vi "run.vi"(8 "error in (no error)":errorcluster, 11 "canon_m3 in":refnum<class "protocol_canonM3.lvclass">) -> (0 "error out":errorcluster, 3 "canon_m3 out":refnum<class "protocol_canonM3.lvclass">)   [LabVIEW 2015, in "protocol_canonM3.lvclass"]
uses:
  protocol_canonM3.lvclass
  protocol_Generic/Protocol_Generic.lvclass
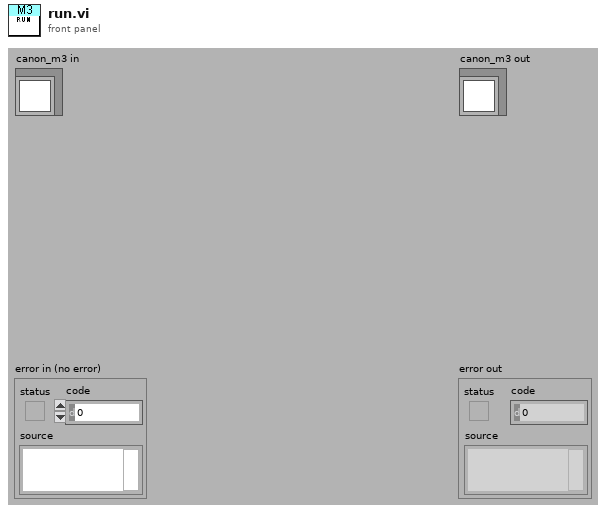
[diagram p1: front panel]
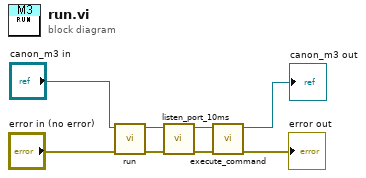
[diagram p0: block diagram]
diagram:
  n1 = call-parent "run.vi"("error in (no error)"="error in (no error)", "Protocol_Generic in"="canon_m3 in") -> ("error out"=w5:errorcluster, "Protocol_Generic out"=w6:refnum<class "protocol_canonM3.lvclass">)  [unwired: 8 in]
  n2 = call-dynamic "listen_port_10ms.vi"("error in (no error)"=w5, "canon_m3 in"=w6) -> ("error out"=w2:errorcluster, "canon_m3 out"=w4:refnum<class "protocol_canonM3.lvclass">)  [unwired: 8 in]
  n3 = call-dynamic "execute_command.vi"("error in (no error)"=w2, "canon_m3 in"=w4) -> ("error out"=→"error out":errorcluster, "canon_m3 out"=→"canon_m3 out":refnum<class "protocol_canonM3.lvclass">)  [unwired: 8 in]
